vi "set_id_mapped.vi"(10 "ID":i32, 11 "Volumes in":refnum<class "CLZ Comics.lvclass">) -> (3 "Volumes out":refnum<class "CLZ Comics.lvclass">)   [LabVIEW 2024, in "CLZ_to_ComicVine.lvlib" / "CLZ Comics.lvclass"]
uses:
  CLZ Comics.lvclass
  CLZ Comics.lvclass/CLZ Comics.ctl
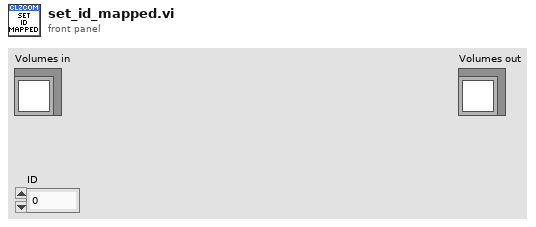
[diagram p1: front panel]
types:
  T1 = typedef "CLZ_to_ComicVine.lvlib/CLZ Comics.lvclass/volume--cluster.ctl" = cluster{"id":i32, "name":string, "issue set":set{string}, "matched":bool}
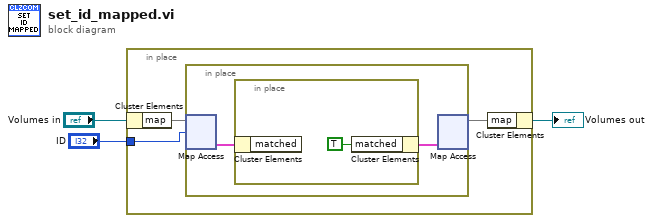
[diagram p0: block diagram]
diagram:
  n1 = in-place {
    in-place-border: "ID" -> [w5]
    n2 = in-place-cluster #1("Volumes in") -> ("map"=w6:map{i32, T1})
    n3 = in-place {
      n4 = in-place-map #2(w6, w5) -> (w8:T1)  [unwired: 1 in, 1 out]
      n5 = in-place {
        n6 = in-place-cluster #3(w8) -> ()  [unwired: 1 out]
        n7 = in-place-cluster #3("matched"=TRUE) -> (w7:T1)
      }
      n8 = in-place-map #2(w7) -> (w4:map{i32, T1})  [unwired: 1 in, 2 out]
    }
    n9 = in-place-cluster #1("map"=w4) -> (→"Volumes out":refnum<class "CLZ Comics.lvclass">)
  }
